vi "Example Panel.vi"   [LabVIEW 2015]
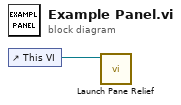
[diagram p0: block diagram]
diagram:
  n1 = control-ref of="This VI"() -> (w1:refnum<vi>)
  n2 = call "Launch Pane Relief.vi"("VI in"=w1) -> ()  [unwired: 9 in, 2 out]
